vi "Robot Systems.vi"(11 "input cluster":T1) -> ()   [LabVIEW 2015]
uses:
  Joystick/ControlsToCommands.ctl
  Robot Global Data.vi
panel:
  in  "Speed":dbl=0.14
  in  "Time":dbl=0.25
  out "What to do":string
  in  "Done 2":bool
  in  "Done":bool
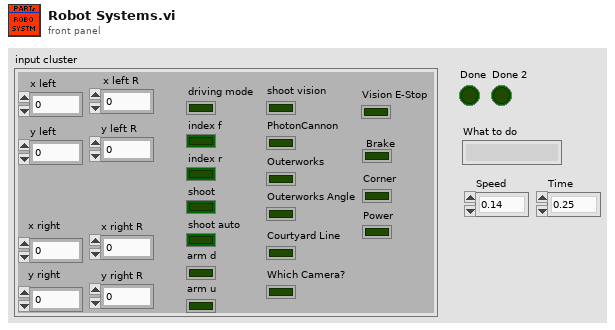
[diagram p1: front panel]
types:
  T1 = typedef "ControlsToCommands.ctl" = cluster{"x left":dbl, "y left":dbl, "x right":dbl, "y right":dbl, "driving mode":bool, "index f":bool, "index r":bool, "shoot":bool, "shoot auto":bool, "arm d":bool, "arm u":bool, "shoot vision":bool, "PhotonCannon":bool, "Outerworks":bool, "Outerworks Angle":bool, "Courtyard Line":bool, "Which Camera?":bool, "Vision E-Stop":bool, "x left R":dbl, "y left R":dbl, "x right R":dbl, "y right R":dbl, "Brake":bool, "Corner":bool, "Power":bool}
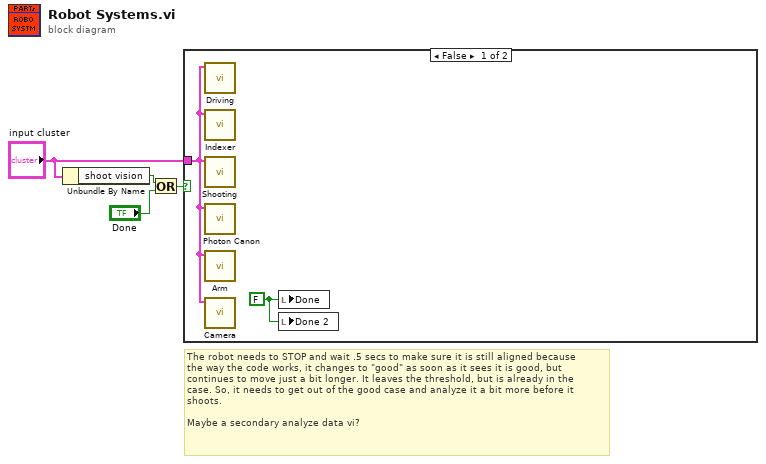
[diagram p0: block diagram]
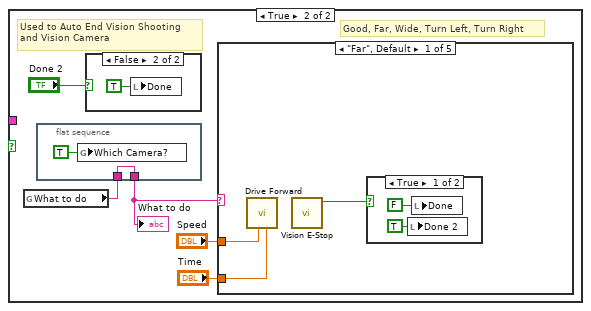
[diagram p2: hidden frame]
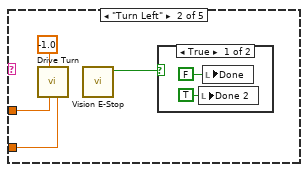
[diagram p4: hidden frame]
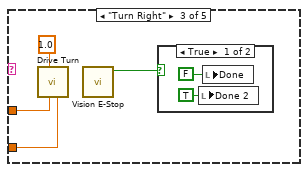
[diagram p6: hidden frame]
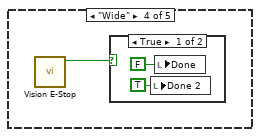
[diagram p8: hidden frame]
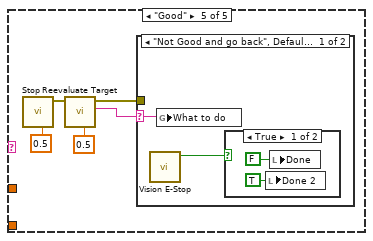
[diagram p10: hidden frame]
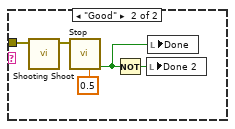
[diagram p12: hidden frame]
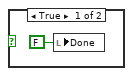
[diagram p13: hidden frame]
diagram:
  # "The robot needs to STOP and wait .5 secs to make sure it is still aligned because \nthe way the code works, it changes to \"good\" as soon as it sees it is good, but \ncontinues to move just a bit longer. It leaves the threshold, but is already in the \ncase. So, it needs to get out of the good case and analyze it a bit more before it \nshoots.\n\nMaybe a secondary analyze data vi?"
  n1 = Unbundle By Name("input cluster") -> ("shoot vision"=w2:bool)
  n2 = Or(x=w2, y="Done") -> (x .or. y?=w1:bool)
  n3 = case shown="False" w1 {
    tunnel: "input cluster" -> [w6 _]
    frame False {
      w5 = FALSE ("Done")
      n4 = call "Driving.vi"("input cluster"=w6) -> ()  [unwired: 11 in]
      n5 = call "Indexer.vi"("input cluster"=w6) -> ()  [unwired: 11 in]
      n6 = call "Shooting.vi"("input cluster"=w6) -> ()  [unwired: 11 in]
      n7 = call "Photon Canon.vi"("input cluster"=w6) -> ()  [unwired: 11 in]
      n8 = call "Arm.vi"("input cluster"=w6) -> ()  [unwired: 11 in]
      n9 = call "Camera.vi"("input cluster"=w6) -> ()  [unwired: 11 in]
      n10 = local write "Done"(w5) -> ()
      n11 = local write "Done 2"(w5) -> ()
    }
    frame True {
      # "Good, Far, Wide, Turn Left, Turn Right"
      # "Used to Auto End Vision Shooting \nand Vision Camera"
      n12 = global read "Robot Global Data.vi" "What to do"() -> (w10:string)
      n13 = flat-sequence {
        tunnel: w10 -> [w46]
        tunnel: [w46] -> w9
        frame #0 {
          n14 = global write "Robot Global Data.vi" "Which Camera?"(TRUE ("Which Camera?")) -> ()
        }
      }
      n15 = case shown="False" "Done 2" {
        frame True {
          n16 = local write "Done"(FALSE ("Done")) -> ()
        }
        frame False {
          n17 = local write "Done"(TRUE ("Done")) -> ()
        }
      }
      n18 = case shown="\"Far\", Default" w9 {
        tunnel: "Speed" -> [w14 w19 w25 _ _]
        tunnel: "Time" -> [w13 w18 w24 _ _]
        frame "Far", Default {
          n19 = call "Drive Forward.vi"("Time"=w13, "Speed"=w14) -> ()  [unwired: 9 in, 1 out]
          n20 = call "Vision E-Stop.vi"() -> ("E-Stop"=w12:bool)  [unwired: 11 in]
          n21 = case shown="True" w12 {
            frame True {
              n22 = local write "Done 2"(TRUE ("Done")) -> ()
              n23 = local write "Done"(FALSE ("Done")) -> ()
            }
            frame False {
            }
          }
        }
        frame "Turn Left" {
          n24 = call "Drive Turn.vi"("Time"=w18, "Speed"=w19, "Direction"=-1.0) -> ()  [unwired: 8 in, 1 out]
          n25 = call "Vision E-Stop.vi"() -> ("E-Stop"=w20:bool)  [unwired: 11 in]
          n26 = case shown="True" w20 {
            frame True {
              n27 = local write "Done 2"(TRUE ("Done")) -> ()
              n28 = local write "Done"(FALSE ("Done")) -> ()
            }
            frame False {
            }
          }
        }
        frame "Turn Right" {
          n29 = call "Drive Turn.vi"("Time"=w24, "Speed"=w25, "Direction"=1.0) -> ()  [unwired: 8 in, 1 out]
          n30 = call "Vision E-Stop.vi"() -> ("E-Stop"=w26:bool)  [unwired: 11 in]
          n31 = case shown="True" w26 {
            frame True {
              n32 = local write "Done 2"(TRUE ("Done")) -> ()
              n33 = local write "Done"(FALSE ("Done")) -> ()
            }
            frame False {
            }
          }
        }
        frame "Wide" {
          n34 = call "Vision E-Stop.vi"() -> ("E-Stop"=w29:bool)  [unwired: 11 in]
          n35 = case shown="True" w29 {
            frame True {
              n36 = local write "Done 2"(TRUE ("Done")) -> ()
              n37 = local write "Done"(FALSE ("Done")) -> ()
            }
            frame False {
            }
          }
        }
        frame "Good" {
          n38 = call "Stop.vi"("Time"=0.5) -> ("error out"=w35:errorcluster)  [unwired: 9 in, 1 out]
          n39 = call "Reevaluate Target.vi"("Delay Time (s)"=0.5 ("Time"), "error in (no error)"=w35) -> ("What to do"=w33:string, "error out (no error)"=w32:errorcluster)  [unwired: 8 in]
          n40 = case shown="\"Not Good and go back\", Default" w33 {
            selector: w33 -> [w38 _]
            tunnel: w32 -> [_ w45]
            frame "Not Good and go back", Default {
              n41 = call "Vision E-Stop.vi"() -> ("E-Stop"=w37:bool)  [unwired: 11 in]
              n42 = global write "Robot Global Data.vi" "What to do"(w38) -> ()
              n43 = case shown="True" w37 {
                frame True {
                  n44 = local write "Done 2"(TRUE ("Done")) -> ()
                  n45 = local write "Done"(FALSE ("Done")) -> ()
                }
                frame False {
                }
              }
            }
            frame "Good" {
              n46 = call "Shooting Shoot.vi"("error in (no error)"=w45) -> ("error out"=w43:errorcluster)  [unwired: 10 in]
              n47 = call "Stop.vi"("Time"=0.5, "error in"=w43) -> ("Done"=w41:bool)  [unwired: 8 in, 1 out]
              n48 = Not(x=w41) -> (.not. x?=w42:bool)
              n49 = local write "Done 2"(w42) -> ()
              n50 = local write "Done"(w41) -> ()
            }
          }
        }
      }
      "What to do" <- w9
    }
  }
